vi "Calibrate Camera.vi"() -> (0 "error out":errorcluster)   [LabVIEW 2020]
uses:
  g_ar_toolkit.common/Camera Parameters.ctl
  g_ar_toolkit.common/Camera Matrix.ctl
  g_ar_toolkit.common/Camera Distortion Coefficients.ctl
  g_ar_toolkit.common/Pose.ctl
  g_ar_toolkit.common/rvec.ctl
  g_ar_toolkit.common/tvec.ctl
  g_ar_toolkit.feature_detection/Chessboard Corner Info.ctl
  g_ar_toolkit.common/Image Size (Integer).ctl
  g_ar_toolkit.common/Object Point (Float).ctl
  g_ar_toolkit.image/CreateEmptyImageGreyscale.vi
  g_ar_toolkit.image/ReadImageFileGreyscale.vi
  g_ar_toolkit.feature_detection/FindChessboardCornersGreyscale.vi
  g_ar_toolkit.image/CreateEmptyImageGreyscale.vi/6598b9e0-8a08-46f5-91fd-ca1b87217137.vi
  g_ar_toolkit.image/ReadImageFileGreyscale.vi/4c855a9e-1811-4d12-9194-a11a862286e6.vi
  g_ar_toolkit.feature_detection/FindChessboardCornersGreyscale.vi/ca99938f-1423-42fb-b653-ffd1f73e2bb5.vi
  <vilib>/Utility/error.llb/Error Cluster From Error Code.vi
  g_ar_toolkit.common/Termination Criteria/Get Values.vi
  g_ar_toolkit.common/Termination Criteria/Termination Criteria.lvclass
  g_ar_toolkit.feature_detection/g_ar_toolkit.feature_detection.lvlib
  g_ar_toolkit.image/g_ar_toolkit.image.lvlib
  g_ar_toolkit.common/g_ar_toolkit.common.lvlib
  g_ar_toolkit.ar/g_ar_toolkit.ar.lvlib
panel:
  out "RMS Error":dbl[](array[numeric])
  out "Poses":T1[](array[typedef])
  out "Camera Parameters":T4
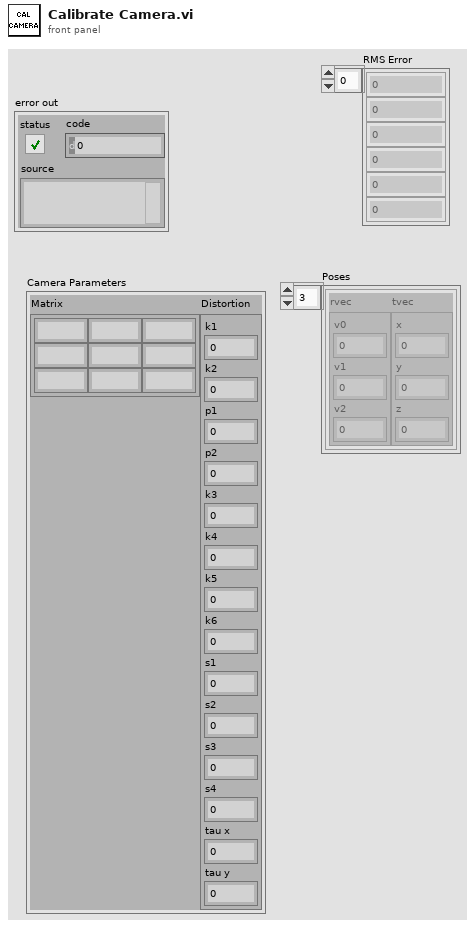
[diagram p1: front panel]
types:
  T1 = typedef "g_ar_toolkit.common.lvlib/Pose.ctl" = cluster{"rvec":T2, "tvec":T3}
  T2 = typedef "g_ar_toolkit.common.lvlib/rvec.ctl" = cluster{"v0":dbl, "v1":dbl, "v2":dbl}
  T3 = typedef "g_ar_toolkit.common.lvlib/tvec.ctl" = cluster{"x":dbl, "y":dbl, "z":dbl}
  T4 = typedef "g_ar_toolkit.common.lvlib/Camera Parameters.ctl" = cluster{"Matrix":T5, "Distortion":T6}
  T5 = typedef "g_ar_toolkit.common.lvlib/Camera Matrix.ctl" = cluster{"m 0,0":dbl, "m 0,1":dbl, "m 0,2":dbl, "m 1,0":dbl, "m 1,1":dbl, "m 1,2":dbl, "m 2,0":dbl, "m 2,1":dbl, "m 2,2":dbl}
  T6 = typedef "g_ar_toolkit.common.lvlib/Camera Distortion Coefficients.ctl" = cluster{"k1":dbl, "k2":dbl, "p1":dbl, "p2":dbl, "k3":dbl, "k4":dbl, "k5":dbl, "k6":dbl, "s1":dbl, "s2":dbl, "s3":dbl, "s4":dbl, "tau x":dbl, "tau y":dbl}
  T7 = typedef "g_ar_toolkit.common.lvlib/Image Size (Integer).ctl" = cluster{"Width":u16, "Height":u16}
  T8 = typedef "g_ar_toolkit.feature_detection.lvlib/Chessboard Corner Info.ctl" = cluster{"Points Per Row":u8, "Points Per Col":u8}
  T9 = cluster{"Points Per Row":i32, "Points Per Col":i32}
  T10 = typedef "g_ar_toolkit.common.lvlib/Object Point (Float).ctl" = cluster{"x":dbl, "y":dbl, "z":dbl}
  T11 = typedef "g_ar_toolkit.common.lvlib/Image Point (Float).ctl" = cluster{"x":dbl, "y":dbl}
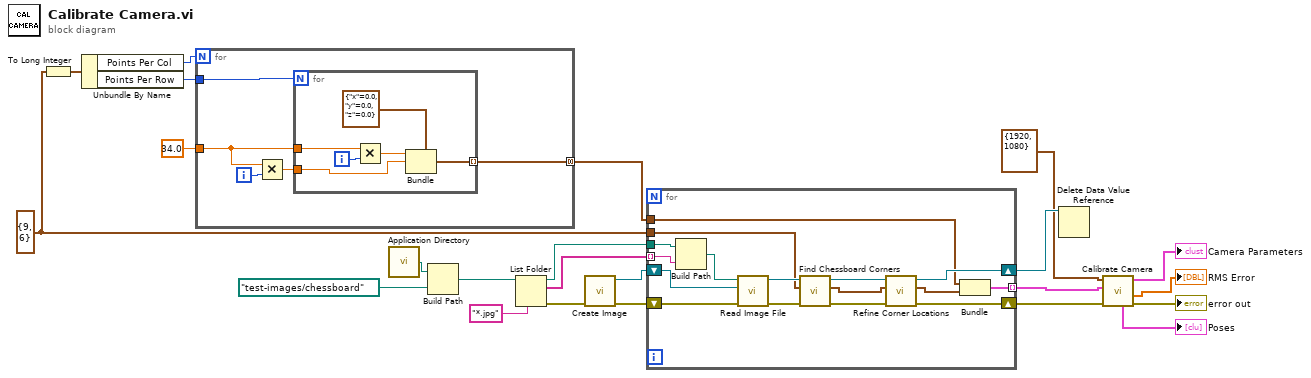
[diagram p0: block diagram]
diagram:
  w13 = T8 {"Points Per Row"=9, "Points Per Col"=6} ("Chessboard Corners Info")
  n1 = To Long Integer(number=w13) -> (32bit integer=w8:T9)
  n2 = Unbundle By Name(w8) -> ("Points Per Col"=w12:i32, "Points Per Row"=w11:i32)
  n3 = for {
    N: w12 -> [_]
    tunnel: w11 -> [w28]
    tunnel: 34.0 -> [w26]
    tunnel: [w24] -> w9 mode=concatenating
    i -> [w27]
    n4 = Multiply(x=w26, y=w27) -> (x*y=w25:dbl)
    n5 = for {
      N: w28 -> [_]
      tunnel: w26 -> [w34]
      tunnel: w25 -> [w30]
      tunnel: [w29] -> w24 mode=indexing
      i -> [w33]
      n6 = Multiply(x=w34, y=w33) -> (x*y=w31:dbl)
      n7 = Bundle(cluster=T10 {"x"=0.0, "y"=0.0, "z"=0.0} ("Object Point"), "x"=w31, "y"=w30) -> (w29:T10)  [unwired: 1 in]
    }
  }
  n8 = call <vilib>:"Application Directory.vi"() -> ("Application Directory"=w20:path)
  n9 = Build Path(base path=w20, name or relative path=path "test-images/chessboard") -> (appended path=w18:path)
  n10 = List Folder(path=w18, pattern="*.jpg") -> (path out=w17:path, filenames=w15:string[], error out=w16:errorcluster)  [unwired: 2 in, 1 out]
  n11 = call-poly "Create Image.vi"("error in (no error)"=w16) -> ("error out"=w22:errorcluster, "New Greyscale Image"=w23:refnum<data-value>)  [unwired: 9 in]
  n12 = for {
    tunnel: w17 -> [w46]
    tunnel: w15 -> [w45] mode=indexing
    shift-right: [w43] -> w7
    shift-left: w22 -> [w48]
    shift-right: [w42] -> w14
    shift-left: w23 -> [w49]
    tunnel: w13 -> [w41]
    tunnel: w9 -> [w40]
    tunnel: [w39] -> w5 mode=indexing
    n13 = Build Path(base path=w46, name or relative path=w45) -> (appended path=w44:path)
    n14 = call-poly "Read Image File.vi"("error in (no error)"=w48, "Greyscale Image Destination"=w49, "Filepath"=w44) -> ("error out"=w47:errorcluster, "Greyscale Image Destination (duplicate)"=w50:refnum<data-value>)  [unwired: 7 in]
    n15 = call-poly "Find Chessboard Corners.vi"("error in (no error)"=w47, "Chessboard Corners Info"=w41, "Greyscale Image"=w50) -> ("error out"=w37:errorcluster, "Points"=w36:T11[], "Greyscale Image (Duplicate)"=w38:refnum<data-value>)  [unwired: 6 in]
    n16 = call "Refine Corner Locations.vi"("error in (no error)"=w37, "Points in"=w36, "Greyscale Image"=w38) -> ("error out"=w43:errorcluster, "Points out"=w35:T11[], "Greyscale Image (Duplicate)"=w42:refnum<data-value>)  [unwired: 6 in]
    n17 = Bundle(w40, "Points out"=w35) -> (w39:cluster{T10[], "Points out":T11[]})  [unwired: 1 in]
  }
  n18 = Delete Data Value Reference(data value reference=w14) -> ()  [unwired: 1 in, 2 out]
  n19 = call "Calibrate Camera.vi"("error in (no error)"=w7, "Point Correspondences"=w5, "Image Size"=T7 {"Width"=1920, "Height"=1080}) -> ("error out"=→"error out":errorcluster, "RMS Error"=→"RMS Error":dbl[], "Camera Parameters"=→"Camera Parameters":T4, "Poses"=→"Poses":T1[])  [unwired: 5 in]
